vi "HW_Set_SYNC_on_ECU_2.vi"(8 "error in (no error)":errorcluster, 10 "IO parameters cluster":T1, 11 "All Port Info":T3={"Type"=enum."Serial (VISA)", "Serial Port"="", "IP Address"="0.0.0.0"}) -> (0 "error out":errorcluster, 3 "Message":string)   [LabVIEW 2018, in "HW Interaction.lvlib"]
uses:
  HW Interaction.lvlib
  Public API/Typedefs/CTL_Port_connection_type.ctl
  SubVi's/Controls/CTL_IO_params_cluster.ctl
  Common_Resources.lvlib
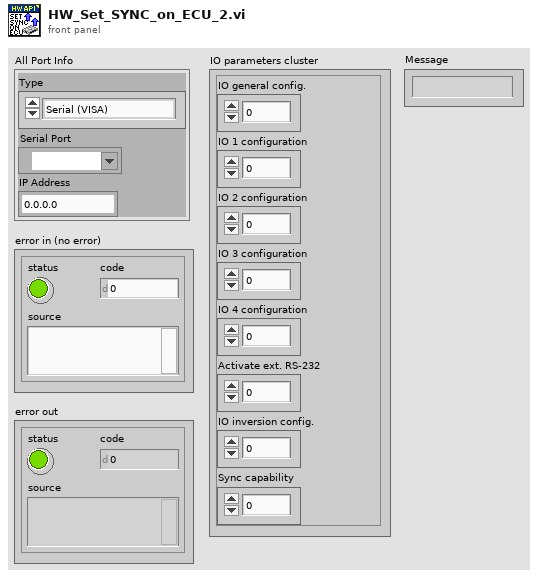
[diagram p1: front panel]
types:
  T1 = typedef "Common_Resources.lvlib/CTL_IO_params_cluster.ctl" = cluster{"IO general config.":u16, "IO 1 configuration":u16, "IO 2 configuration":u16, "IO 3 configuration":u16, "IO 4 configuration":u16, "Activate ext. RS-232":u16, "IO inversion config.":u16, "Sync capability":u8}
  T2 = typedef "HW Interaction.lvlib/CTL_Port_connection_type.ctl" = enum16{"Serial (VISA)", "TCP/IP"}
  T3 = cluster{"Type":T2, "Serial Port":refnum<visa-resource-name>, "IP Address":string}
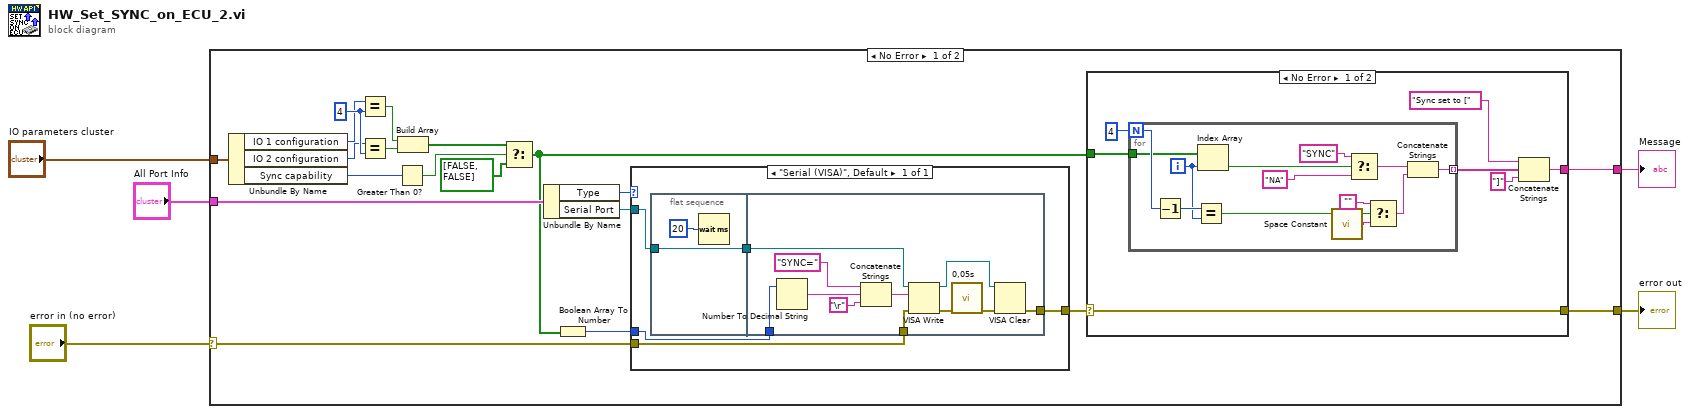
[diagram p0: block diagram]
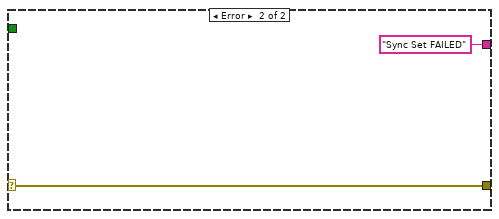
[diagram p2: hidden frame]
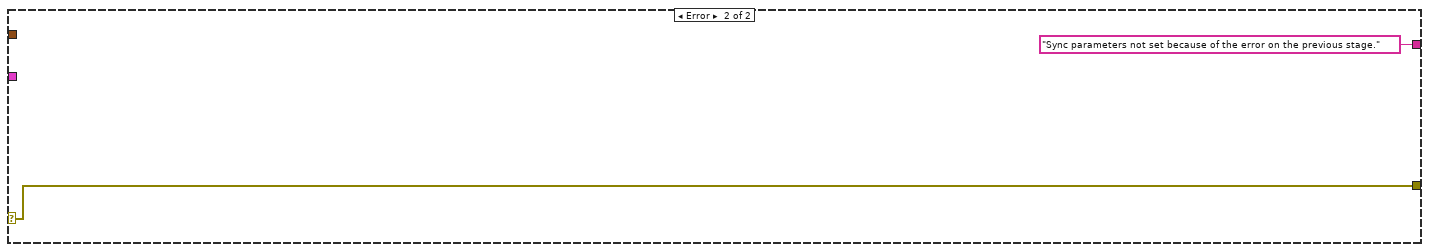
[diagram p3: hidden frame]
diagram:
  n1 = case shown="No Error" "error in (no error)" {
    selector: "error in (no error)" -> [w21 w66]
    tunnel: [w12 w66] -> w5
    tunnel: "All Port Info" -> [w24 _]
    tunnel: "IO parameters cluster" -> [w20 _]
    tunnel: [w13 "Sync parameters not set because of the error on the previous stage."] -> w1
    frame No Error {
      w19 = u16 4
      n2 = Unbundle By Name(w20) -> ("IO 1 configuration"=w18:u16, "IO 2 configuration"=w17:u16, "Sync capability"=w6:u8)
      n3 = Equal?(x=w18, y=w19) -> (x = y?=w16:bool)
      n4 = Equal?(x=w17, y=w19) -> (x = y?=w15:bool)
      n5 = Greater Than 0?(x=w6) -> (x > 0?=w11:bool)
      n6 = Build Array(w16, w15) -> (w9:bool[])
      n7 = Select(t=w9, s=w11, f=bool[] [FALSE, FALSE]) -> (s? t:f=w8:bool[])
      n8 = Unbundle By Name(w24) -> ("Type"=w23:T2, "Serial Port"=w22:refnum<visa-resource-name>)
      n9 = Boolean Array To Number(Boolean array=w8) -> (number=w10:u32)
      n10 = case shown="\"Serial (VISA)\", Default" w23 {
        tunnel: [w50] -> w14
        tunnel: w22 -> [w49]
        tunnel: w21 -> [w48]
        tunnel: w10 -> [w47]
        frame "Serial (VISA)", Default {
          n11 = flat-sequence {
            tunnel: w49 -> [w53]
            tunnel: [w53] -> w51
            tunnel: [w64] -> w50
            tunnel: w47 -> [w57]
            tunnel: w48 -> [w59]
            tunnel: w51 -> [w60]
            frame #0 {
              n12 = Wait (ms)(milliseconds to wait=u32 20) -> ()  [unwired: 1 out]
            }
            frame #1 {
              n13 = Number To Decimal String(number=w57) -> (decimal integer string=w56:string)  [unwired: 1 in]
              n14 = Concatenate Strings("SYNC=" ("f"), w56, "\r") -> (w61:string)
              n15 = VISA Write(VISA resource name=w60, write buffer=w61, error in (no error)=w59) -> (VISA resource name out=w54:refnum<visa-resource-name>, error out=w63:errorcluster)  [unwired: 1 out]
              n16 = call "0,05s"("error in (no error)"=w63) -> ("error out"=w55:errorcluster)  [unwired: 10 in]
              n17 = VISA Clear(VISA resource name=w54, error in (no error)=w55) -> (error out=w64:errorcluster)  [unwired: 1 out]
            }
          }
        }
      }
      n18 = case shown="No Error" w14 {
        selector: w14 -> [w31 w46]
        tunnel: [w31 w46] -> w12
        tunnel: [w29 "Sync Set FAILED"] -> w13
        tunnel: w8 -> [w26 _]
        frame No Error {
          n19 = for {
            N: 4 -> [w44]
            tunnel: [w42] -> w28 mode=indexing
            tunnel: w26 -> [w37]
            i -> [w36]
            n20 = Decrement(x=w44) -> (x-1=w43:i32)
            n21 = Equal?(x=w43, y=w36) -> (x = y?=w41:bool)
            n22 = Index Array(array=w37, index=w36) -> (element=w35:bool)
            n23 = call <vilib>:"Space Constant.vi"() -> ("String"=w38:string)
            n24 = Select(t="SYNC", s=w35, f="NA") -> (s? t:f=w32:string)
            n25 = Select(t="", s=w41, f=w38) -> (s? t:f=w40:string)
            n26 = Concatenate Strings(w32, w40) -> (w42:string)
          }
          n27 = Concatenate Strings("Sync set to [", w28, "]" ("string")) -> (w29:string)
        }
        frame Error {
        }
      }
    }
    frame Error {
    }
  }
  "error out" <- w5
  "Message" <- w1
